vi "Main Page.vi"(8 "error in (no error)":errorcluster, 11 "Node Ptr":T1 format="%.0x") -> (0 "error out":errorcluster)   [LabVIEW 2017, in "VeriStand Web Service Demo System Explorer.lvlib"]
uses:
  VeriStand Web Service Demo System Explorer.lvlib
  <vilib>/NI Veristand/Custom Device API/Custom Device Item Ref.ctl
  <vilib>/NI/NI VeriStand Advanced SysDef API/_SubVIs/SysDef.Property.Get.String.vi
  <vilib>/NI/NI VeriStand Advanced SysDef API/_SubVIs/SysDef.Property.Set.String.vi
  <vilib>/NI VeriStand/Custom Device API/Custom Device API.lvlib
  <vilib>/NI/NI VeriStand Advanced SysDef API/SysDef API/Advanced System Definition.lvlib
panel:
  in  "Queue Name":string
  out "Version":string
  in  "SHDocVw.IWebBrowser":refnum<k7>(container)
  in  "Specific Header":cluster{"Section Name":string}={"Section Name"="Custom Device Item Settings"}
  in  "General Header":cluster{"Section Name":string}={"Section Name"="General Custom Device Settings"}
  in  "Description":string
  in  "Name":string
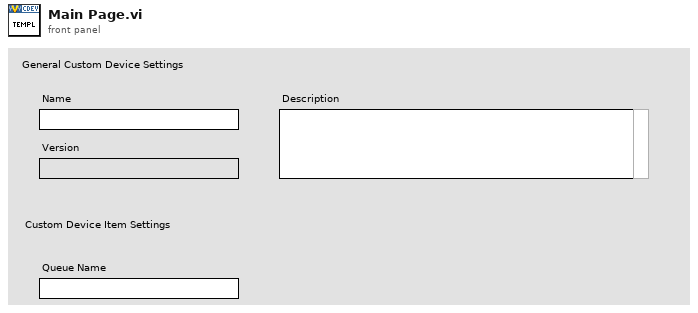
[diagram p1: front panel]
types:
  T1 = typedef "Custom Device API.lvlib/Custom Device Item Ref.ctl" = u64
  T2 = typedef "Custom Device API.lvlib/Custom Device Item Info.ctl" = cluster{"Name":string, "Is Channel":bool, "GUID":string, "Is Waveform":bool}
  T3 = typedef "Custom Device API.lvlib/Custom Device Commands.ctl" = enum16{"Default", "Item renamed", "Shutdown", "Dynamic button pressed"}
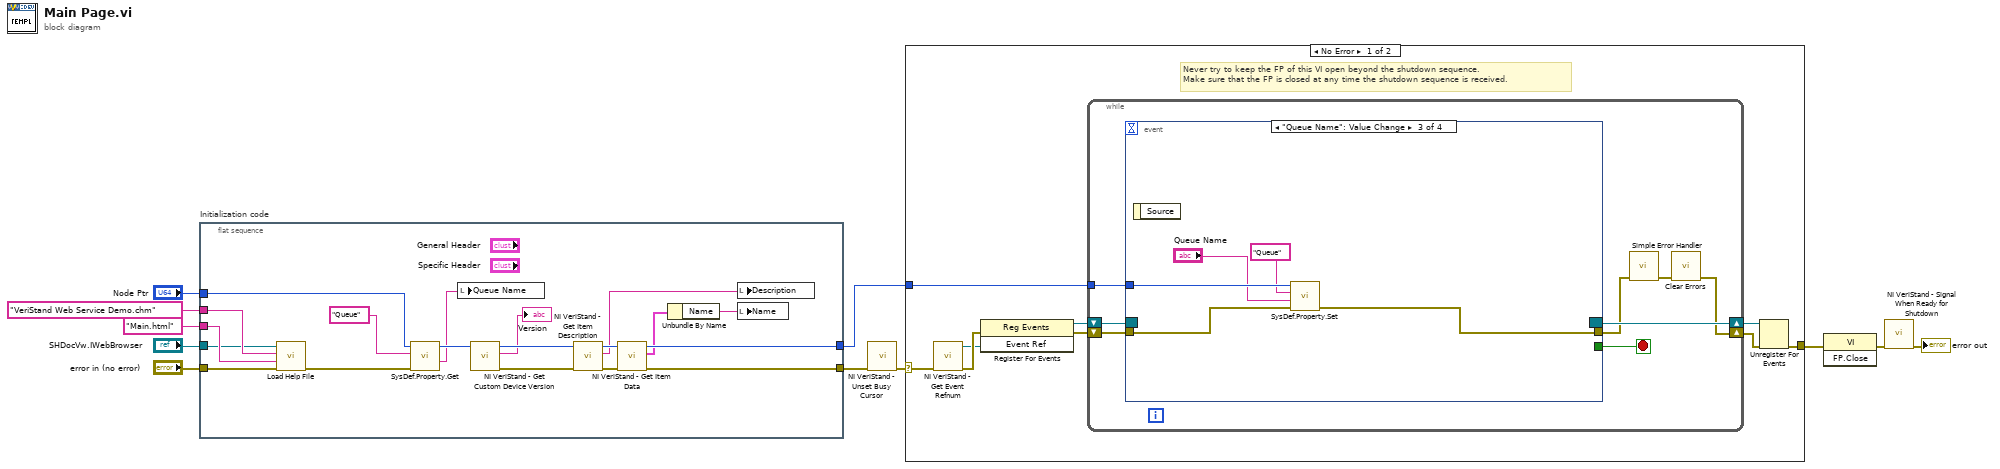
[diagram p0: block diagram]
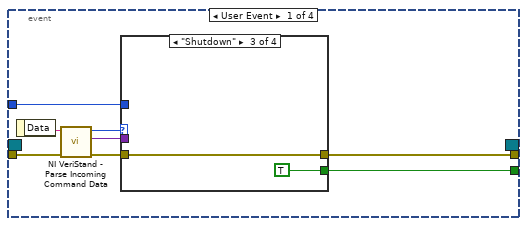
[diagram p2: hidden frame]
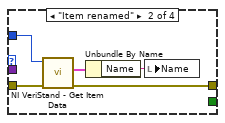
[diagram p4: hidden frame]
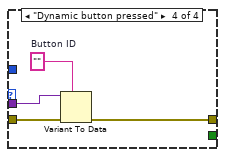
[diagram p5: hidden frame]
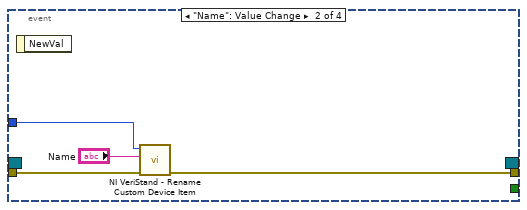
[diagram p6: hidden frame]
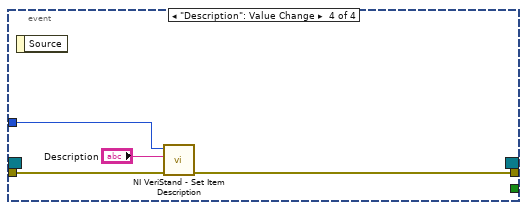
[diagram p7: hidden frame]
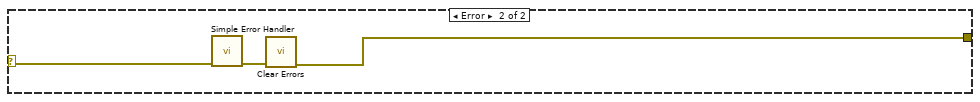
[diagram p8: hidden frame]
diagram:
  n1 = flat-sequence "Initialization code" {
    tunnel: "error in (no error)" -> [w22]
    tunnel: "Node Ptr" -> [w15]
    tunnel: [w26] -> w7
    tunnel: [w30] -> w4
    tunnel: "SHDocVw.IWebBrowser" -> [w19]
    tunnel: "Main.html" ("HTML File") -> [w21]
    tunnel: "VeriStand Web Service Demo.chm" ("CD_CHM_FileName") -> [w20]
    frame #0 {
      n2 = call "Load Help File.vi"("error in (no error)"=w22, "HTML File to Load"=w21, "Main CHM File"=w20, "Browser"=w19) -> ("error out"=w16:errorcluster)  [unwired: 7 in]
      n3 = call-poly <vilib>:"SysDef.Property.Get.vi"("error in (no error)"=w16, "Property Name"="Queue", "nodeID"=w15) -> ("Value out"=w12:string, "nodeID out"=w14:u64)  [unwired: 5 in, 2 out]
      n4 = local write "Queue Name"(w12) -> ()
      n5 = call <vilib>:"NI VeriStand - Get Custom Device Version.vi"("Device Ref in"=w14) -> ("error out"=w25:errorcluster, "Value"=→"Version":string, "Device Ref out"=w24:T1)  [unwired: 8 in]
      n6 = call <vilib>:"NI VeriStand - Get Item Description.vi"("error in (no error)"=w25, "Item Ref in"=w24) -> ("error out"=w28:errorcluster, "Description"=w17:string, "Item Ref out"=w29:T1)  [unwired: 7 out]
      n7 = call <vilib>:"NI VeriStand - Get Item Data.vi"("error in (no error)"=w28, "Item Ref in"=w29) -> ("error out"=w26:errorcluster, "Item Info"=w27:T2, "Item Ref out"=w30:T1)  [unwired: 7 out]
      n8 = Unbundle By Name(w27) -> ("Name"=w18:string)
      n9 = local write "Description"(w17) -> ()
      n10 = local write "Name"(w18) -> ()
    }
  }
  n11 = call <vilib>:"NI VeriStand - Unset Busy Cursor.vi"("error in (no error)"=w7) -> ("error out"=w6:errorcluster)  [unwired: 10 out]
  n12 = case shown="No Error" w6 {
    selector: w6 -> [w31 w83]
    tunnel: [w36 w81] -> w11
    tunnel: w4 -> [w32 _]
    frame No Error {
      # "Never try to keep the FP of this VI open beyond the shutdown sequence.\nMake sure that the FP is closed at any time the shutdown sequence is received."
      n13 = call <vilib>:"NI VeriStand - Get Event Refnum.vi"("error in (no error)"=w31) -> ("error out"=w39:errorcluster, "Event Ref"=w35:refnum<user-event>)  [unwired: 9 out]
      n14 = register-events(error in=w39, w35) -> (reference out=w33:refnum<event-registration>, error out=w34:errorcluster)  [unwired: 1 in]
      n15 = while {
        tunnel: w32 -> [w43]
        shift-right: [w40] -> w37
        shift-left: w34 -> [w46]
        shift-right: [w47] -> w38
        shift-left: w33 -> [w45]
        stop <- w44 stop-if-true
        n16 = event shown="[2] \"Queue Name\": Value Change" {
          selector: w45 -> [_ _ _ _]
          dyn-events: [_ _ _ _] -> w47
          timeout: _ -> [_ _ _ _]
          tunnel: w46 -> [w55 w71 w73 w79]
          tunnel: [w51 _ _ _] -> w44
          tunnel: [w50 w70 w72 w78] -> w42
          tunnel: w43 -> [w49 w69 w76 w80]
          event User Event {
            n17 = event-data() -> ("Data"=w54:string)  [unwired: 1 out]
            n18 = call <vilib>:"NI VeriStand - Parse Incoming Command Data.vi"("error in (no error)"=w55, "Incoming data"=w54) -> ("error out"=w53:errorcluster, "Outgoing data"=w48:variant, "Action"=w52:T3)  [unwired: 7 out]
            n19 = case shown="\"Shutdown\"" w52 {
              tunnel: w53 -> [w56 w61 w62 w67]
              tunnel: [_ _ TRUE _] -> w51
              tunnel: [w56 w58 w62 w64] -> w50
              tunnel: w49 -> [_ w60 _ _]
              tunnel: w48 -> [_ _ _ w66]
              frame "Default", Default {
              }
              frame "Item renamed" {
                n20 = call <vilib>:"NI VeriStand - Get Item Data.vi"("error in (no error)"=w61, "Item Ref in"=w60) -> ("error out"=w58:errorcluster, "Item Info"=w59:T2)  [unwired: 8 out]
                n21 = Unbundle By Name(w59) -> ("Name"=w57:string)
                n22 = local write "Name"(w57) -> ()
              }
              frame "Shutdown" {
              }
              frame "Dynamic button pressed" {
                w65 = ""  # Button ID
                n23 = Variant To Data(error in=w67, type=w65, Variant=w66) -> (error out=w64:errorcluster)  [unwired: 1 out]
              }
            }
          }
          event "Name": Value Change {
            n24 = event-data() -> ()  [unwired: 2 out]
            n25 = call <vilib>:"NI VeriStand - Rename Custom Device Item.vi"("error in (no error)"=w71, "New Name"="Name", "Item Ref in"=w69) -> ("error out"=w70:errorcluster)  [unwired: 1 in, 7 out]
          }
          event "Queue Name": Value Change {
            n26 = event-data() -> ()  [unwired: 2 out]
            n27 = call-poly <vilib>:"SysDef.Property.Set.vi"("error in (no error)"=w73, "Value"="Queue Name", "Property Name"="Queue", "nodeID"=w76) -> ("error out"=w72:errorcluster)  [unwired: 6 in, 1 out]
          }
          event "Description": Value Change {
            n28 = event-data() -> ()  [unwired: 2 out]
            n29 = call <vilib>:"NI VeriStand - Set Item Description.vi"("error in (no error)"=w79, "Description"="Description", "Item Ref in"=w80) -> ("error out"=w78:errorcluster)  [unwired: 8 out]
          }
        }
        n30 = call <vilib>:"Simple Error Handler.vi"("error in (no error)"=w42) -> ("error out"=w41:errorcluster)  [unwired: 1 in, 7 out]
        n31 = call <vilib>:"Clear Errors.vi"("error in (no error)"=w41) -> ("error out"=w40:errorcluster)  [unwired: 1 in, 5 out]
      }
      n32 = Unregister For Events(event registration refnum=w38, error in=w37) -> (error out=w36:errorcluster)
    }
    frame Error {
      n33 = call <vilib>:"Simple Error Handler.vi"("error in (no error)"=w83) -> ("error out"=w82:errorcluster)  [unwired: 1 in, 7 out]
      n34 = call <vilib>:"Clear Errors.vi"("error in (no error)"=w82) -> ("error out"=w81:errorcluster)  [unwired: 1 in, 5 out]
    }
  }
  n35 = invoke class="VI" method="FP.Close"(error in=w11) -> (error out=w10:errorcluster)  [unwired: 2 in, 2 out]
  n36 = call <vilib>:"NI VeriStand - Signal When Ready for Shutdown.vi"("error in (no error)"=w10) -> ("error out"=→"error out":errorcluster)  [unwired: 10 out]
